vi "init.vi"(8 "error in":errorcluster, 10 "TBM module configuration in":refnum<class "TBM module configuration.lvclass">, 11 "Scaling runtime in":refnum<class "Scaling runtime.lvclass">) -> (0 "error out":errorcluster, 1 "data allocations":T1, 2 "execution settings":T4, 3 "Scaling runtime out":refnum<class "Scaling runtime.lvclass">)   [LabVIEW 2013, in "Scaling runtime.lvclass"]
doc: "Provides an interface for initializing a module at runtime. While this interface performs no operations, a child should provide an override which may open any necessary references or sessions, allocate necessary memory, and perform any final configuration validataion before providing the full configuration <b>execution data</b> to the calling process."
uses:
  Scaling runtime.lvclass
  <vilib>/NI/Tag Bus Module Framework/channel/TBM channel.lvclass
  <vilib>/NI/Tag Bus Module Framework/runtime/TBM module execution interface.lvclass
  configuration/Scaling configuration.lvclass
  <vilib>/NI/Tag Bus Module Framework/module configuration/TBM module configuration.lvclass
  <vilib>/NI/Tag Bus Module Framework/runtime/execution settings.ctl
  <vilib>/NI/Tag Bus Module Framework/channel/data tables.ctl
  <vilib>/NI/Tag Bus/dictionary/data dictionary.lvclass
  <vilib>/NI/Tag Bus/dictionary table pair.ctl
  <vilib>/NI/Tag Bus/tag bus.lvlib
  <vilib>/NI/Tag Bus/table/data table.ctl
  <vilib>/NI/Tag Bus/table/data table.lvlib
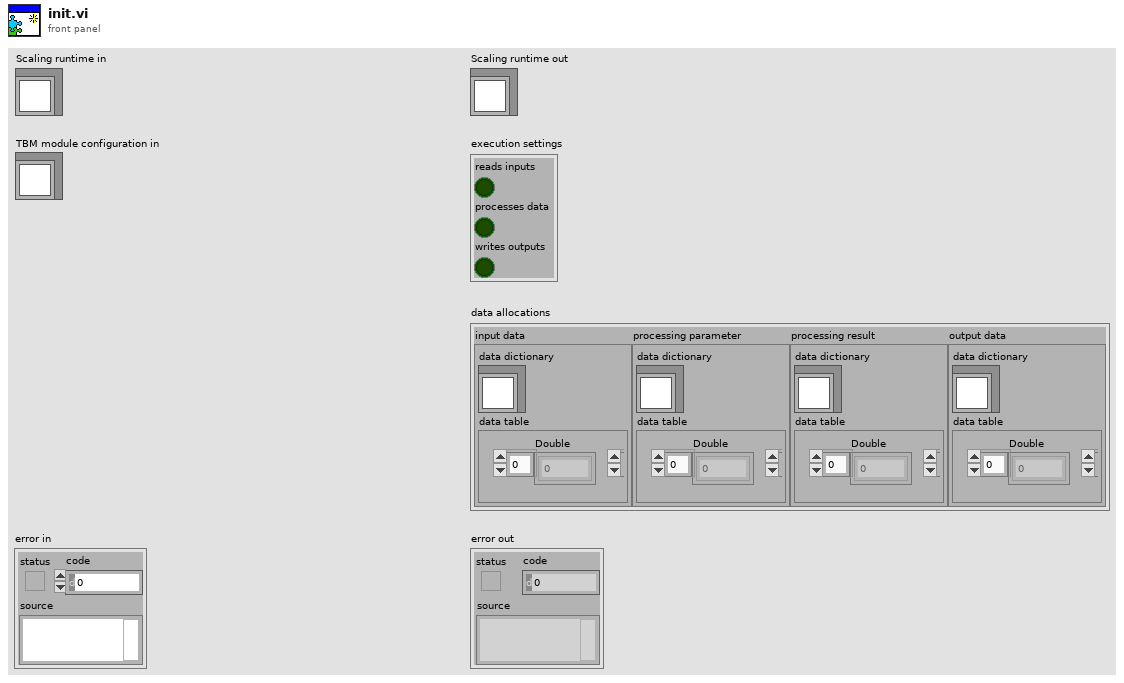
[diagram p1: front panel]
types:
  T1 = typedef "TBM channel.lvclass/data tables.ctl" = cluster{"input data":T2, "processing parameter":T2, "processing result":T2, "output data":T2}
  T2 = typedef "tag bus.lvlib/dictionary table pair.ctl" = cluster{"data dictionary":refnum<class "data dictionary.lvclass">, "data table":T3}
  T3 = typedef "tag bus.lvlib/data table.lvlib/data table.ctl" = cluster{"Double":dbl[], "Single":sgl[], "I64":i64[], "I32":i32[], "I16":i16[], "I8":i8[], "U64":u64[], "U32":u32[], "U16":u16[], "U8":u8[], "Boolean":bool[], "String":string[], "Array of Double":cluster{"DBL Array":dbl[]}[], "Array of Single":cluster{"SGL Array":sgl[]}[], "Array of I64":cluster{"I64 Array":i64[]}[], "Array of I32":cluster{"I32 Array":i32[]}[], "Array of I16":cluster{"I16 Array":i16[]}[], "Array of I8":cluster{"I8 Array":i8[]}[], "Array of U64":cluster{"U64 Array":u64[]}[], "Array of U32":cluster{"U32 Array":u32[]}[], "Array of U16":cluster{"U16 Array":u16[]}[], "Array of U8":cluster{"U8 Array":u8[]}[], "Array of Boolean":cluster{"Boolean Array":bool[]}[], "Array of String":cluster{"String Array":string[]}[]}
  T4 = typedef "TBM module execution interface.lvclass/execution settings.ctl" = cluster{"reads inputs":bool, "processes data":bool, "writes outputs":bool}
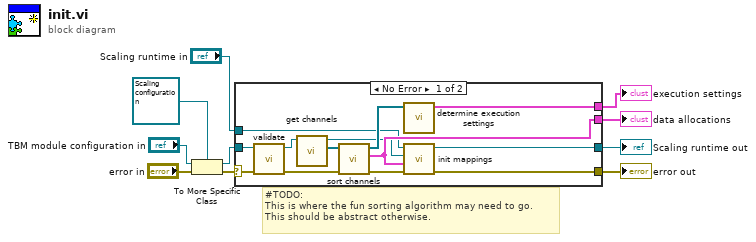
[diagram p0: block diagram]
diagram:
  # "#TODO:\nThis is where the fun sorting algorithm may need to go.\nThis should be abstract otherwise."
  n1 = To More Specific Class(target class=refnum<class "Scaling configuration.lvclass"> refnum ("Synchronous module configuration"), reference="TBM module configuration in", error in="error in") -> (specific class reference=w9:refnum<class "Scaling configuration.lvclass">, error out=w10:errorcluster)
  n2 = case shown="No Error" w10 {
    selector: w10 -> [w20 w24]
    tunnel: w9 -> [w19 _]
    tunnel: "Scaling runtime in" -> [w13 w25]
    tunnel: [w12 w25] -> w4
    tunnel: [w11 w24] -> w3
    tunnel: [w15 _] -> w1
    tunnel: [w23 _] -> w2
    frame No Error {
      n3 = call-dynamic "validate.vi"("error in"=w20, "Scaling configuration in"=w19) -> ("error out"=w21:errorcluster, "Scaling configuration out"=w17:refnum<class "Scaling configuration.lvclass">)  [unwired: 8 in]
      n4 = call-dynamic "get channels.vi"("Scaling configuration in"=w17) -> ("channels"=w18:refnum<class "TBM channel.lvclass">[], "Scaling configuration out"=w14:refnum<class "Scaling configuration.lvclass">)  [unwired: 9 in]
      n5 = call <vilib>:"sort channels.vi"("error in"=w21, "channels in"=w18) -> ("error out"=w16:errorcluster, "data allocations"=w15:T1, "channels out"=w22:refnum<class "TBM channel.lvclass">[])  [unwired: 7 in]
      n6 = call <vilib>:"determine execution settings.vi"("channels"=w22) -> ("execution settings"=w23:T4)  [unwired: 10 in]
      n7 = call "init mappings.vi"("error in (no error)"=w16, "data allocations"=w15, "Scaling configuration"=w14, "Scaling runtime in"=w13) -> ("error out"=w11:errorcluster, "Scaling runtime out"=w12:refnum<class "Scaling runtime.lvclass">)  [unwired: 6 in]
    }
    frame Error {
    }
  }
  "error out" <- w3
  "Scaling runtime out" <- w4
  "execution settings" <- w2
  "data allocations" <- w1
